vi "Voltage Collection (SubVI).vi"(0 "error in (no error)":errorcluster, 1 "Signal Name":string, 11 "data":dynamicdata(waveform)) -> (4 "error out":errorcluster, 6 "?":dbl, 8 "?":dbl format="%0.2f", 10 "?":dynamicdata(graph), 15 "Signals Out":dynamicdata(waveform))   [LabVIEW 2018]
uses:
  <vilib>/express/express shared/transition.llb/Dynamic To Waveform Array.vi
  <vilib>/express/express signal manip/GetorSetDDTAttributes/Set DDT Attributes/SetT0.vi
  <vilib>/express/express shared/transition.llb/Waveform Array To Dynamic.vi
  <vilib>/express/express signal manip/GetorSetDDTAttributes/Set DDT Attributes/Set DDT Properties.xnode
  <vilib>/ptbypt/NI_PtbyPt.lvlib
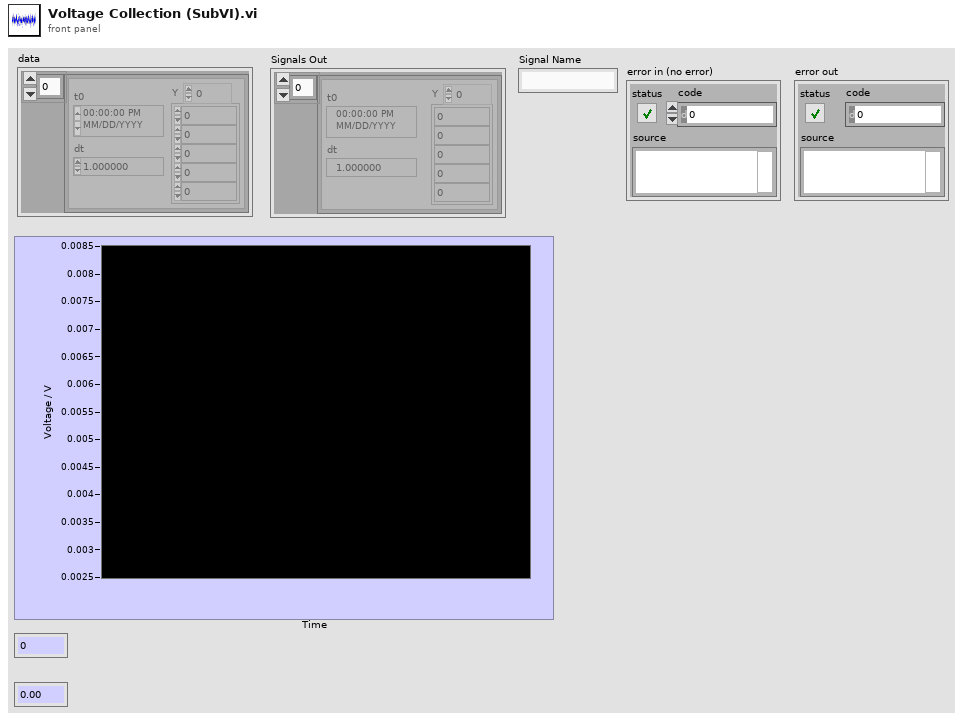
[diagram p1: front panel]
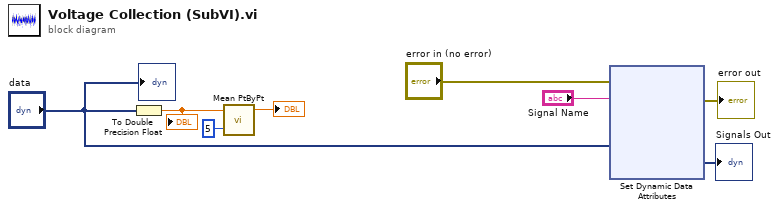
[diagram p0: block diagram]
diagram:
  n1 = To Double Precision Float(number="data") -> (double precision float=w5:dbl)
  "?" <- w5
  n2 = call <vilib>:"Mean PtByPt.vi"("x"=w5, "sample length"=5) -> ("mean"=→"?":dbl)  [unwired: 2 in, 1 out]
  n3 = xnode "Set Dynamic Data Attributes"("Signals In"="data", "error in"="error in (no error)", "Signal Name"="Signal Name") -> ("Signals Out"=→"Signals Out":dynamicdata, "error out"=→"error out":errorcluster)  [unwired: 1 in]
  "?" <- "data"
